vi "multipart_Body_Binary.vi"(8 "error in":errorcluster, 11 "Multpart/Form-Data":T1(array[cluster])) -> (0 "error out":errorcluster, 3 "Multipart Binary Body":string)   [LabVIEW 2016, in "Request.lvclass"]
uses:
  Object Oriented Version/Request/Request.lvclass
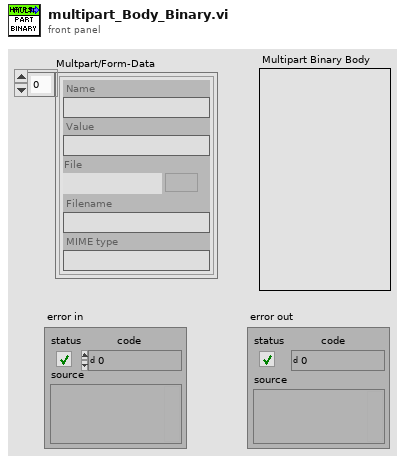
[diagram p1: front panel]
types:
  T1 = cluster{"Name":string, "Value":string, "File":path, "Filename":string, "MIME type":string}[]
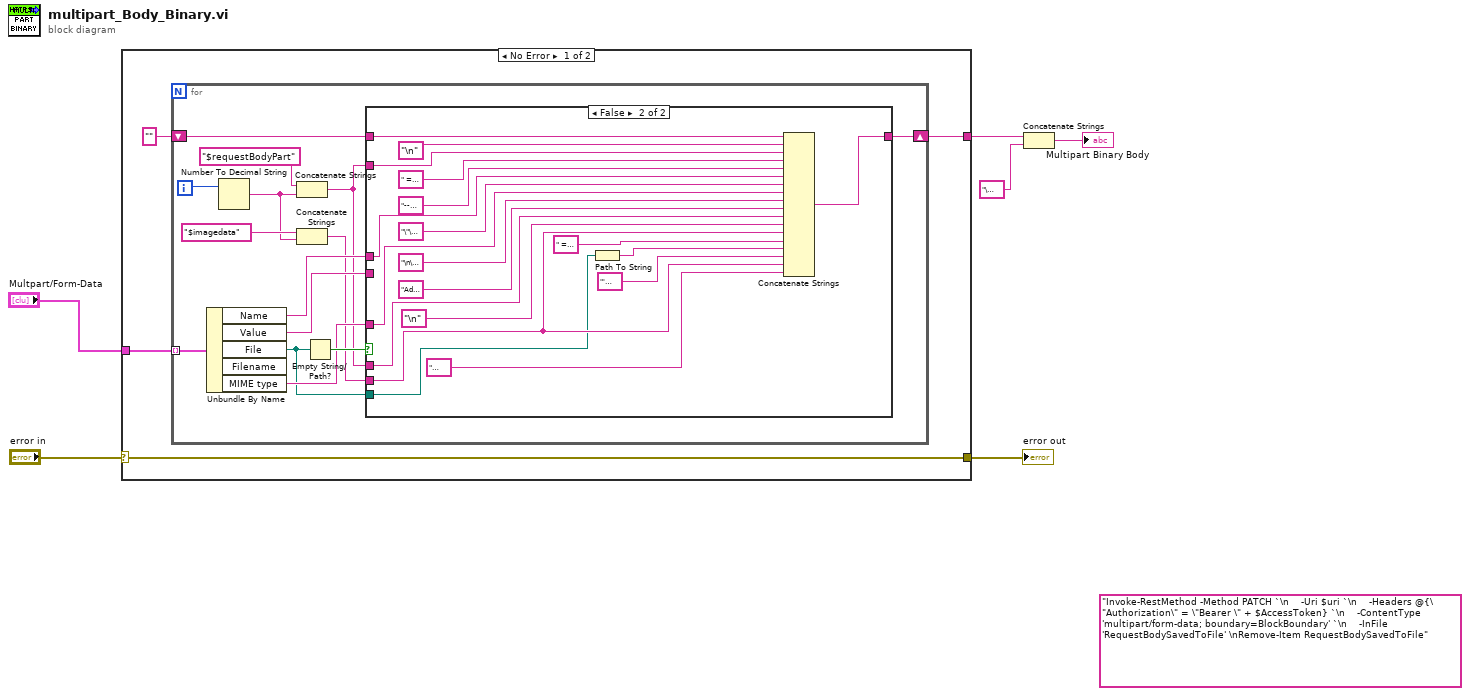
[diagram p0: block diagram]
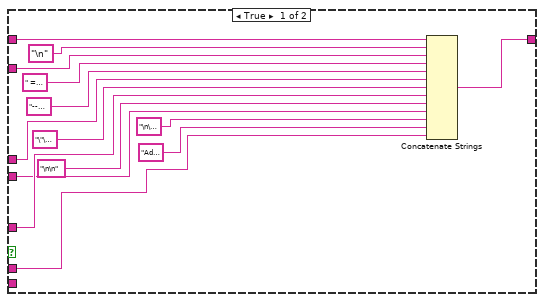
[diagram p2: hidden frame]
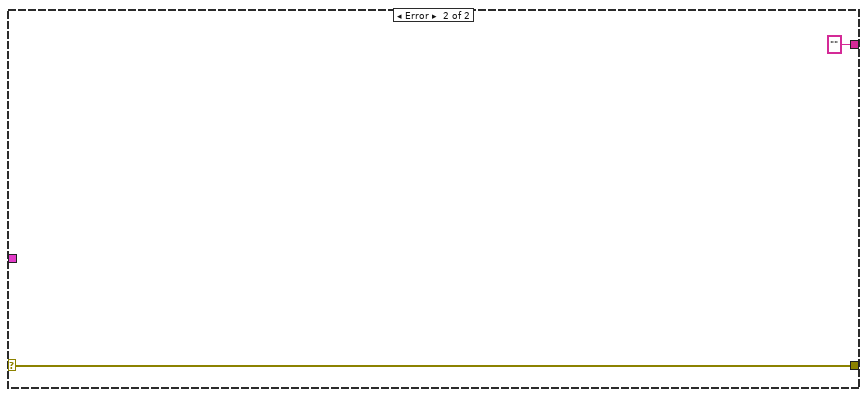
[diagram p3: hidden frame]
diagram:
  (unwired) "Invoke-RestMethod -Method PATCH `\n    -Uri $uri `\n    -Headers @{\"Authorization\" = \"Bearer \" + $AccessToken} `\n    -ContentType 'multipart/form-data; boundary=BlockBoundary' `\n    -InFile 'RequestBodySavedToFile' \nRemove-Item RequestBodySavedToFile"
  n1 = case shown="No Error" "error in" {
    selector: "error in" -> [w7 w58]
    tunnel: "Multpart/Form-Data" -> [w10 _]
    tunnel: [w8 ""] -> w5
    tunnel: [w7 w58] -> w2
    frame No Error {
      n2 = for {
        tunnel: w10 -> [w24] mode=indexing
        shift-right: [w19] -> w8
        shift-left: "" -> [w20]
        i -> [w22]
        n3 = Unbundle By Name(w24) -> ("Name"=w18:string, "Value"=w16:string, "File"=w11:path, "MIME type"=w17:string)  [unwired: 1 out]
        n4 = Number To Decimal String(number=w22) -> (decimal integer string=w13:string)  [unwired: 1 in]
        n5 = Concatenate Strings("$requestBodyPart", w13) -> (w15:string)
        n6 = Concatenate Strings("$imagedata" ("string"), w13) -> (w12:string)
        n7 = Empty String/Path?(string/path=w11) -> (empty?=w23:bool)
        n8 = case shown="False" w23 {
          tunnel: w15 -> [w38 w57]
          tunnel: w20 -> [w36 w55]
          tunnel: [w35 w54] -> w19
          tunnel: w18 -> [w28 w45]
          tunnel: w17 -> [w27 w44]
          tunnel: w16 -> [w26 _]
          tunnel: w15 -> [w25 w41]
          tunnel: w12 -> [_ w40]
          tunnel: w11 -> [_ w39]
          frame True {
            n9 = Concatenate Strings(w36, "\n" ("string"), w38, " = @\"\n" ("string"), "--BlockBoundary\nContent-Disposition:form-data; name=\"", w28, "\"\nContent-Type:" ("string"), w27, "\n\n" ("string"), w26, "\n\n\"@\n" ("string"), "Add-Content 'RequestBodySavedToFile' ", w25) -> (w35:string)
          }
          frame False {
            n10 = Path To String(path=w39) -> (string=w48:string)
            n11 = Concatenate Strings(w55, "\n" ("string"), w57, " = @\"\n" ("string"), "--BlockBoundary\nContent-Disposition:form-data; name=\"", w45, "\"\nContent-Type:" ("string"), w44, "\n\n\"@\n" ("string"), "Add-Content 'RequestBodySavedToFile' ", w41, "\n" ("string"), w40, " = Get-Content '" ("string"), w48, "' -Raw -Encoding Byte\nAdd-Content 'RequestBodySavedToFile' " ("string"), w40, " -Encoding Byte\n" ("string")) -> (w54:string)
          }
        }
      }
    }
    frame Error {
    }
  }
  "error out" <- w2
  n12 = Concatenate Strings(w5, "\n$requestBodySuffix = @\"\n\n--BlockBoundary--\n\"@\nAdd-Content 'RequestBodySavedToFile' $requestBodySuffix") -> (→"Multipart Binary Body":string)
